vi "Untitled 5.vi"(8 "error in":errorcluster) -> (0 "error out":errorcluster, 3 "task out":refnum<k21>)   [LabVIEW 2020]
uses:
  <vilib>/DAQmx/create/channels.llb/DAQmx Create Channel (AI-Bridge).vi
  <vilib>/DAQmx/configure/timing.llb/DAQmx Timing (Sample Clock).vi
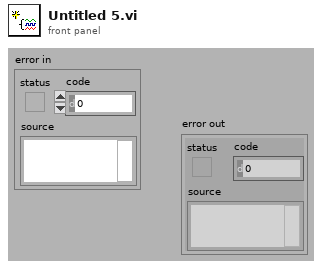
[diagram p1: front panel]
types:
  T1 = cluster{"bridge configuration":i32, "voltage excitation source":i32, "voltage excitation value":dbl, "nominal bridge resistance":dbl}
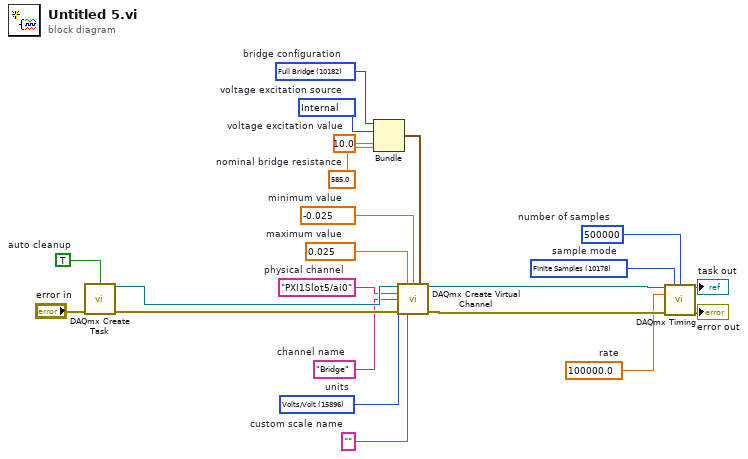
[diagram p0: block diagram]
diagram:
  w1 = 10178 items=["Finite Samples"=10178, "Continuous Samples"=10123, "Hardware Timed Single Point"=12522]  # sample mode
  w2 = 500000  # number of samples
  w3 = 100000.0  # rate
  w7 = 15896 items=["Volts/Volt"=15896, "mVolts/Volt"=15897, "From Custom Scale"=10065]  # units
  w8 = 585.0  # nominal bridge resistance
  w9 = 10.0  # voltage excitation value
  w10 = 10200 items=["None"=10230, "Internal"=10200, "External"=10167]  # voltage excitation source
  w11 = 10182 items=["Full Bridge"=10182, "Half Bridge"=10187, "Quarter Bridge"=10270]  # bridge configuration
  w13 = "Bridge"  # channel name
  w15 = ""  # custom scale name
  w16 = -0.025  # minimum value
  w17 = 0.025  # maximum value
  w18 = "PXI1Slot5/ai0"  # physical channel
  w20 = TRUE  # auto cleanup
  n1 = call <vilib>:"DAQmx Create Task.vi"("auto cleanup"=w20, "error in"="error in") -> ("task out"=w19:refnum<k21>, "error out"=w21:errorcluster)  [unwired: 12 in]
  n2 = Bundle("bridge configuration"=w11, "voltage excitation source"=w10, "voltage excitation value"=w9, "nominal bridge resistance"=w8) -> (w12:T1)  [unwired: 1 in]
  n3 = call-poly <vilib>:"DAQmx Create Virtual Channel.vi"("task in"=w19, "maximum value"=w17, "minimum value"=w16, "bridge information"=w12, "physical channels"=w18, "name to assign"=w13, "units"=w7, "error in"=w21, "custom scale name"=w15) -> ("task out"=w4:refnum<k21>, "error out"=w14:errorcluster)  [unwired: 5 in]
  n4 = call-poly <vilib>:"DAQmx Timing.vi"("task/channels in"=w4, "sample mode"=w1, "samples per channel"=w2, "rate"=w3, "error in"=w14) -> ("task out"=→"task out":refnum<k21>, "error out"=→"error out":errorcluster)  [unwired: 9 in]
